vi "3일차2vi.vi"() -> ()   [LabVIEW 2014]
uses:
  <vilib>/Analysis/NI_AALBase.lvlib
panel:
  out "숫자형":i32
  in  "정지":bool
  out "웨이브폼 그래프":dbl[](graph)
  in  "열거형":enum16{"사인파", "삼각파", "톱니파", "DC신호", "노이즈신호"}(ring)
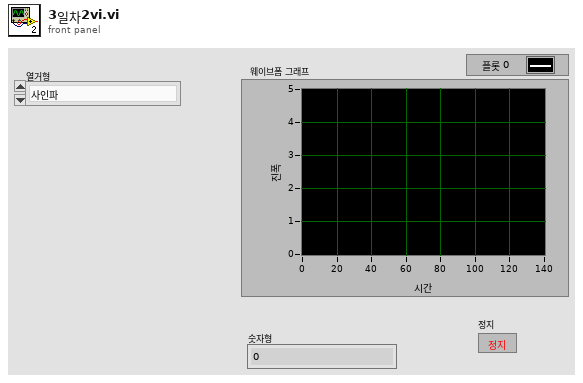
[diagram p1: front panel]
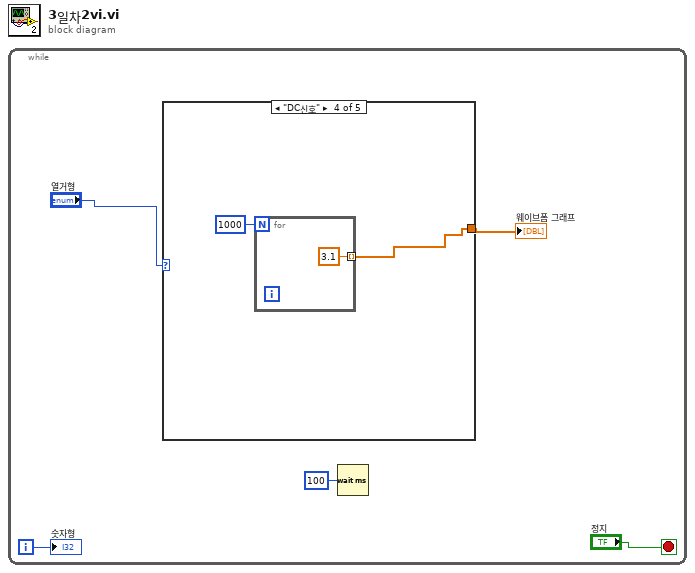
[diagram p0: block diagram]
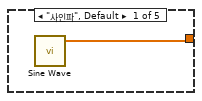
[diagram p2: hidden frame]
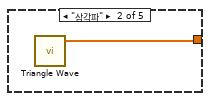
[diagram p3: hidden frame]
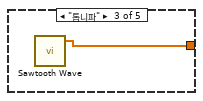
[diagram p4: hidden frame]
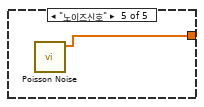
[diagram p5: hidden frame]
diagram:
  n1 = while {
    i -> [w2]
    stop <- "정지" stop-if-true
    n2 = case shown="\"DC신호\"" "열거형" {
      tunnel: [w6 w7 w8 w9 w12] -> w4
      frame "사인파", Default {
        n3 = call <vilib>:"Sine Wave.vi"() -> ("sine wave"=w6:dbl[])  [unwired: 5 in, 2 out]
      }
      frame "삼각파" {
        n4 = call <vilib>:"Triangle Wave.vi"() -> ("triangle wave"=w7:dbl[])  [unwired: 5 in, 2 out]
      }
      frame "톱니파" {
        n5 = call <vilib>:"Sawtooth Wave.vi"() -> ("sawtooth wave"=w8:dbl[])  [unwired: 5 in, 2 out]
      }
      frame "DC신호" {
        n6 = for {
          N: 1000 -> [_]
          tunnel: [3.1] -> w9 mode=indexing
        }
      }
      frame "노이즈신호" {
        n7 = call <vilib>:"Poisson Noise.vi"() -> ("poisson noise"=w12:dbl[])  [unwired: 10 in, 1 out]
      }
    }
    "웨이브폼 그래프" <- w4
    n8 = Wait (ms)(milliseconds to wait=u32 100 ("대기 시간(ms)")) -> ()  [unwired: 1 out]
    "숫자형" <- w2
  }
